vi "Set mode.vi"(8 "error in (no error)":errorcluster, 11 "Motor in":refnum<class "Motor.lvclass">) -> (0 "error out":errorcluster, 3 "Motor out":refnum<class "Motor.lvclass">)   [LabVIEW 2018, in "Motor.lvclass"]
uses:
  Motor.lvclass
  Motor.lvclass/Motor.ctl
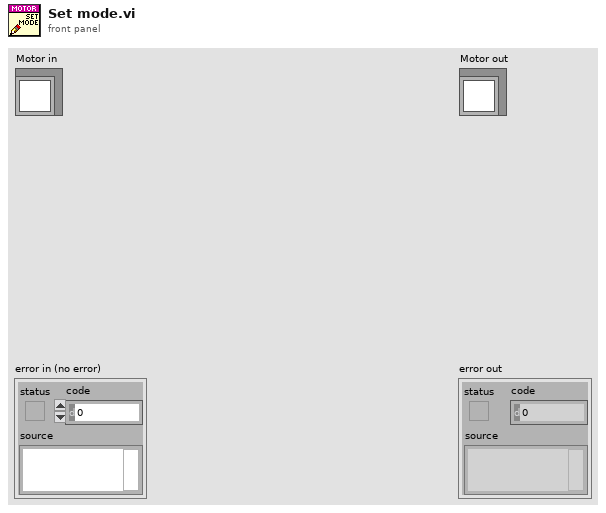
[diagram p1: front panel]
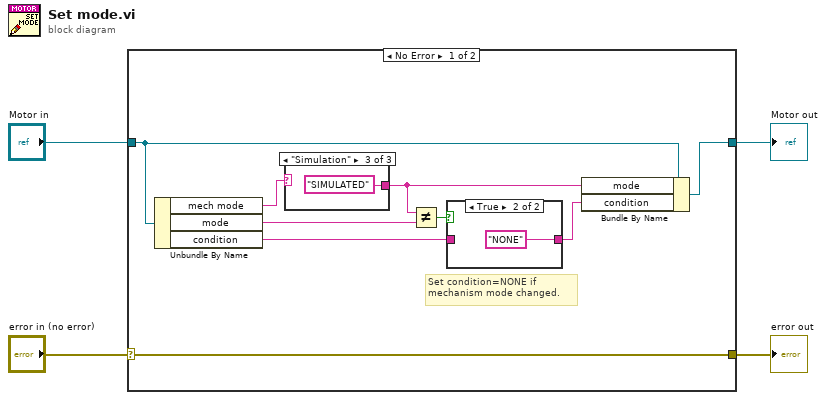
[diagram p0: block diagram]
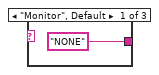
[diagram p3: hidden frame]
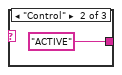
[diagram p4: hidden frame]
diagram:
  n1 = case shown="No Error" "error in (no error)" {
    selector: "error in (no error)" -> [w13 w19]
    tunnel: [w13 w19] -> w3
    tunnel: [w12 w20] -> w1
    tunnel: "Motor in" -> [w11 w20]
    frame No Error {
      # "Set condition=NONE if \nmechanism mode changed."
      n2 = Unbundle By Name(w11) -> ("mech mode"=w6:string, "mode"=w7:string, "condition"=w8:string)
      n3 = case shown="\"Simulation\"" w6 {
        tunnel: ["NONE" "ACTIVE" "SIMULATED"] -> w5
        frame "Monitor", Default {
        }
        frame "Control" {
        }
        frame "Simulation" {
        }
      }
      n4 = Not Equal?(x=w5, y=w7) -> (x != y?=w9:bool)
      n5 = case shown="True" w9 {
        tunnel: [w14 "NONE"] -> w10
        tunnel: w8 -> [w14 _]
        frame False {
        }
        frame True {
        }
      }
      n6 = Bundle By Name(cluster=w11, "mode"=w5, "condition"=w10) -> (w12:refnum<class "Motor.lvclass">)
    }
    frame Error {
    }
  }
  "error out" <- w3
  "Motor out" <- w1
